vi "TEC Server.vi"() -> ()   [LabVIEW 2025]
uses:
  controls/TED4015 Connection.ctl
  controls/TED4015 Status.ctl
  <vilib>/Utility/error.llb/DialogType.ctl
  <vilib>/addons/_JKI Toolkits/State Machine/_JKI_lib_State_Machine.llb/Select State(s)_err__jki_lib_state_machine.vi
  <vilib>/addons/_JKI Toolkits/State Machine/_JKI_lib_State_Machine.llb/Periodic Trigger__ogtk__JKI-SM__jki_lib_state_machine.vi
  <userlib>/_OpenG.lib/comparison/comparison.llb/1D Boolean Array Changed__ogtk.vi
  <userlib>/_OpenG.lib/comparison/comparison.llb/openg_comparison__ogtk.lvlib
panel:
  in  "DiodeNames":string[](array[string])=["InAs", "InGaAs"]
  in  "DiodeNames 2":string[](array[string])
  out "error out":errorcluster {"code" format="%.0x"}
  in  "Tab Control":enum32{"Graph", "Export"}(tab)
  out "TED":waveform(dbl)[](graph)=[{"t0"=timestamp(3845871052.1406174 s since 1904-01-01), "dt"=1.0, "Y"=[23.85494], "attributes"=variant("NI_ChannelName"=variant(string "TED_Temp_0"))}, {"t0"=timestamp(3845871052.1406174 s since 1904-01-01), "dt"=1.0, "Y"=[0.0], "attributes"=variant("NI_ChannelName"=variant(string "TED_Voltage_0"))}, {"t0"=timestamp(3845871052.1406174 s since 1904-01-01), "dt"=1.0, "Y"=[0.001787742], "attributes"=variant("NI_ChannelName"=variant(string "TED_Current_0"))}, {"t0"=timestamp(3845871052.1406174 s since 1904-01-01), "dt"=1.0, "Y"=[21.97219], "attributes"=variant("NI_ChannelName"=variant(string "TED_Temp_1"))}, {"t0"=timestamp(3845871052.1406174 s since 1904-01-01), "dt"=1.0, "Y"=[0.0], "attributes"=variant("NI_ChannelName"=variant(string "TED_Voltage_1"))}, {"t0"=timestamp(3845871052.1406174 s since 1904-01-01), "dt"=1.0, "Y"=[0.00642528], "attributes"=variant("NI_ChannelName"=variant(string "TED_Current_1"))}]
  out "TED_Wfm":T1={"Temp"=[{"t0"=timestamp(3845871052.1406174 s since 1904-01-01), "dt"=1.0, "Y"=[23.85494], "attributes"=variant("NI_ChannelName"=variant(string "TED_Temp_0"))}, {"t0"=timestamp(3845871052.1406174 s since 1904-01-01), "dt"=1.0, "Y"=[21.97219], "attributes"=variant("NI_ChannelName"=variant(string "TED_Temp_1"))}], "Volts"=[{"t0"=timestamp(3845871052.1406174 s since 1904-01-01), "dt"=1.0, "Y"=[0.001787742], "attributes"=variant("NI_ChannelName"=variant(string "TED_Current_0"))}, {"t0"=timestamp(3845871052.1406174 s since 1904-01-01), "dt"=1.0, "Y"=[0.00642528], "attributes"=variant("NI_ChannelName"=variant(string "TED_Current_1"))}], "Amps"=[{"t0"=timestamp(3845871052.1406174 s since 1904-01-01), "dt"=1.0, "Y"=[0.0], "attributes"=variant("NI_ChannelName"=variant(string "TED_Voltage_0"))}, {"t0"=timestamp(3845871052.1406174 s since 1904-01-01), "dt"=1.0, "Y"=[0.0], "attributes"=variant("NI_ChannelName"=variant(string "TED_Voltage_1"))}]}
  in  "TEC On":bool[](array[boolean])=[FALSE, FALSE]
  in  "TED Status":T2[](array[typedef])=[{"Output"=FALSE, "SetPoint"=-65.00001, "Temperature"=23.85494, "Current"=0.0, "Voltage"=0.001787742, "CableTrip"=FALSE, "TransducerTrip"=FALSE, "OverTemp"=FALSE}, {"Output"=FALSE, "SetPoint"=-65.00001, "Temperature"=21.97219, "Current"=0.0, "Voltage"=0.00642528, "CableTrip"=FALSE, "TransducerTrip"=FALSE, "OverTemp"=FALSE}]
  in  "TED4015s":T3[](array[typedef])=[{"VISA resource name"="TED-1", "Connected"=FALSE, "Serial Number"=""}, {"VISA resource name"="TED-2", "Connected"=FALSE, "Serial Number"=""}]
  in  "Exit":bool
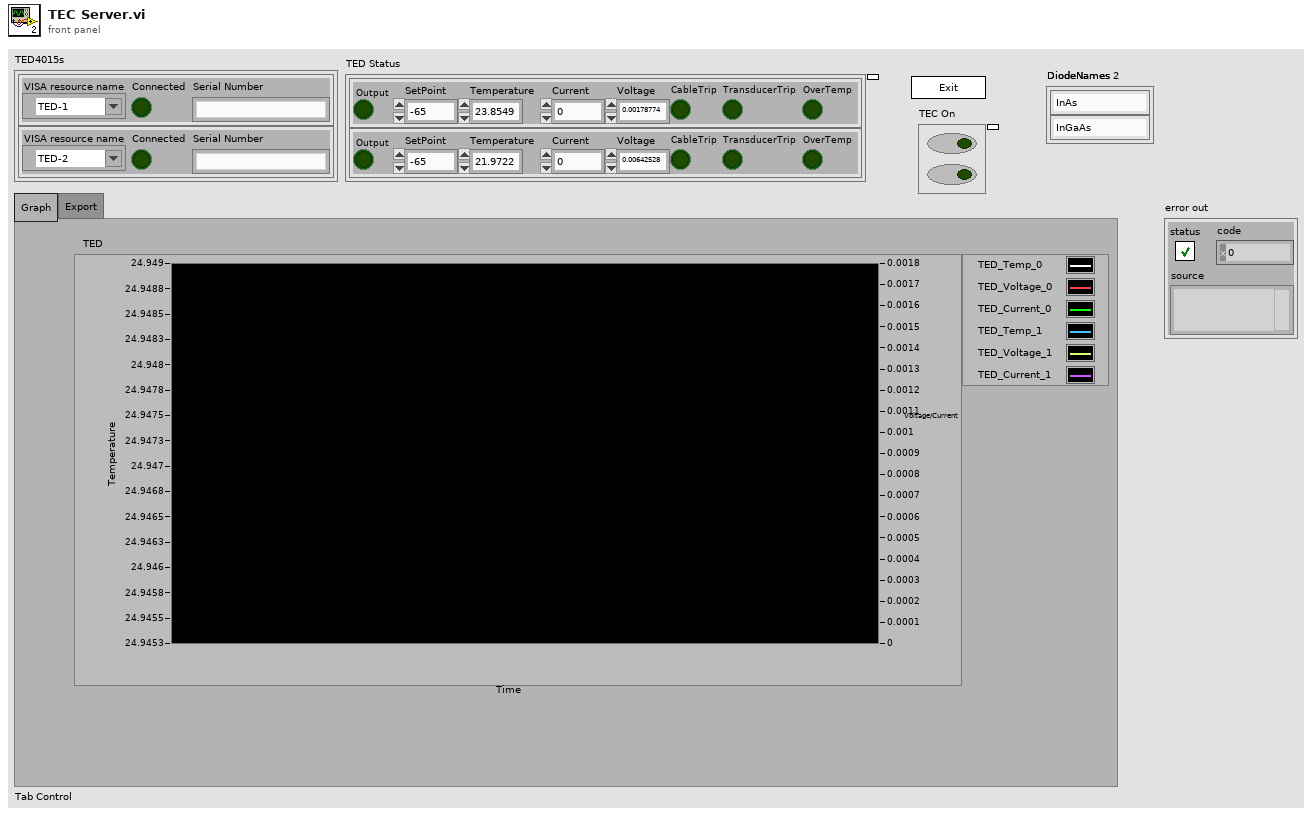
[diagram p1: front panel]
types:
  T1 = cluster{"Temp":waveform(dbl)[], "Volts":waveform(dbl)[], "Amps":waveform(dbl)[]}
  T2 = typedef "TED4015 Status.ctl" = cluster{"Output":bool, "SetPoint":dbl, "Temperature":dbl, "Current":dbl, "Voltage":dbl, "CableTrip":bool, "TransducerTrip":bool, "OverTemp":bool}
  T3 = typedef "TED4015 Connection.ctl" = cluster{"VISA resource name":refnum<visa-resource-name>, "Connected":bool, "Serial Number":string}
  T4 = enum32{"invalid app kind", "Development System", "Run Time System", "Student Edition", "Embedded LabVIEW", "Evaluation", "Custom"}
  T5 = enum32{"Invalid", "Standard", "Closed", "Hidden", "Minimized", "Maximized"}
  T6 = cluster{"Core":cluster{"Current VI Reference":refnum<vi>, "Close Panel on Exit?":bool}, "TED4015s":T3[], "TED Status":T2[], "TED_Wfm":cluster{"Temp":waveform(dbl)[], "Volts":waveform(dbl)[], "Amps":waveform(dbl)[]}}
  T7 = typedef "DialogType.ctl" = u16
  T8 = cluster{"Current VI Reference":refnum<vi>, "Close Panel on Exit?":bool}
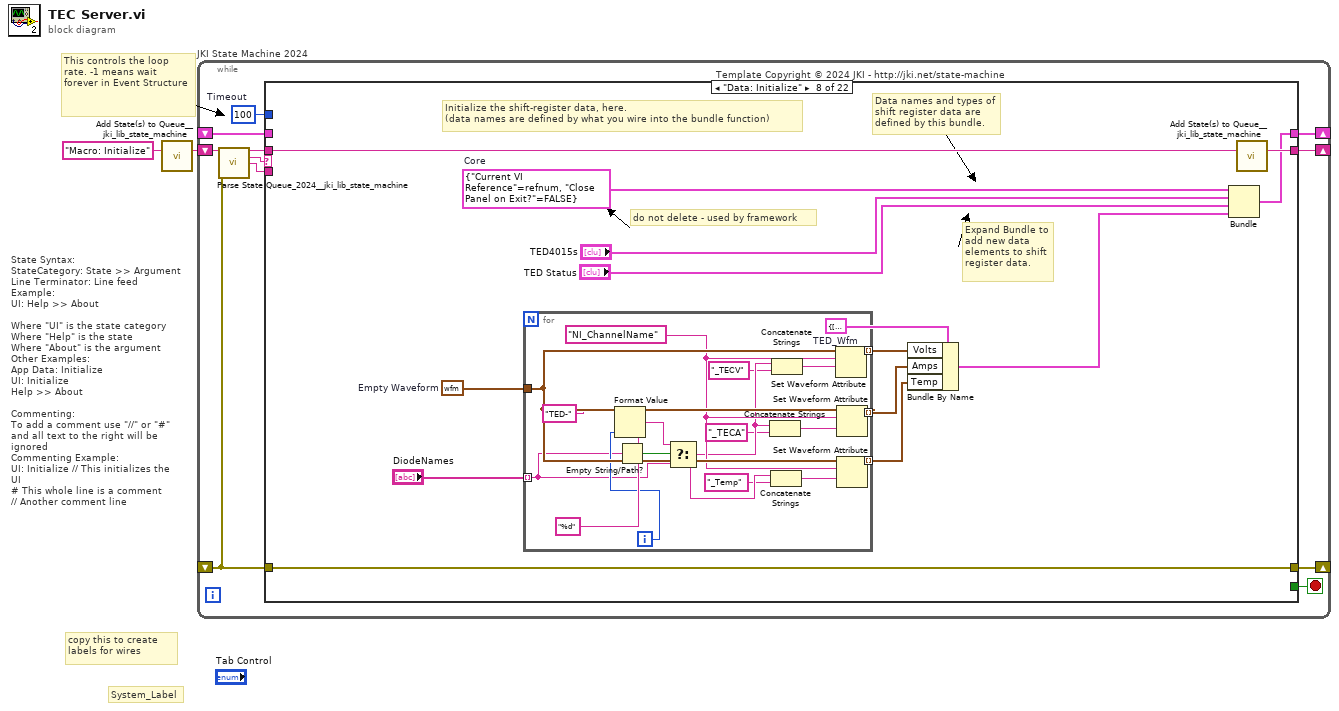
[diagram p0: block diagram]
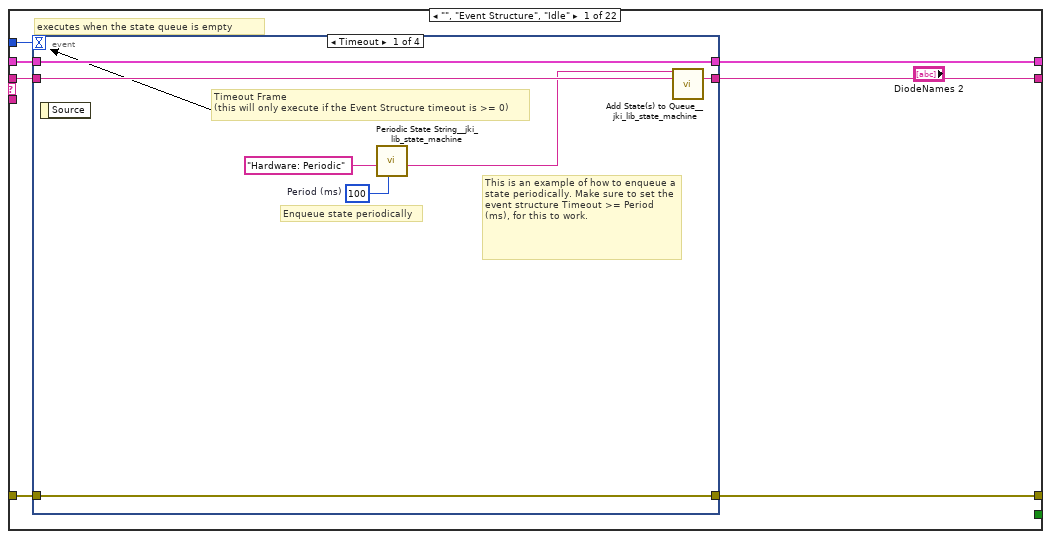
[diagram p2: hidden frame]
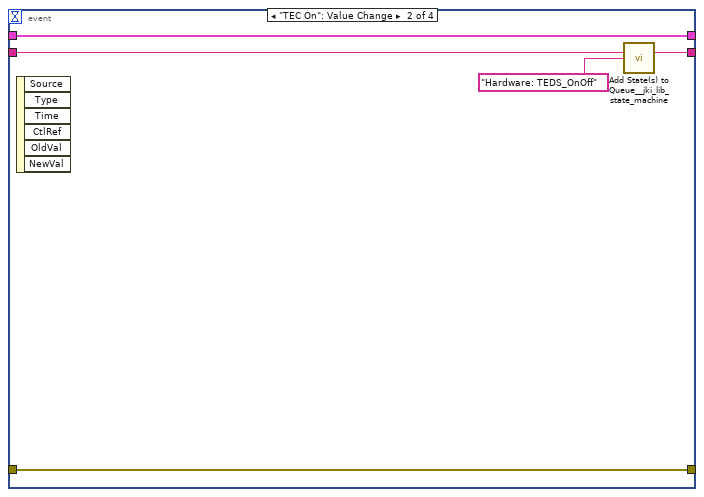
[diagram p3: hidden frame]
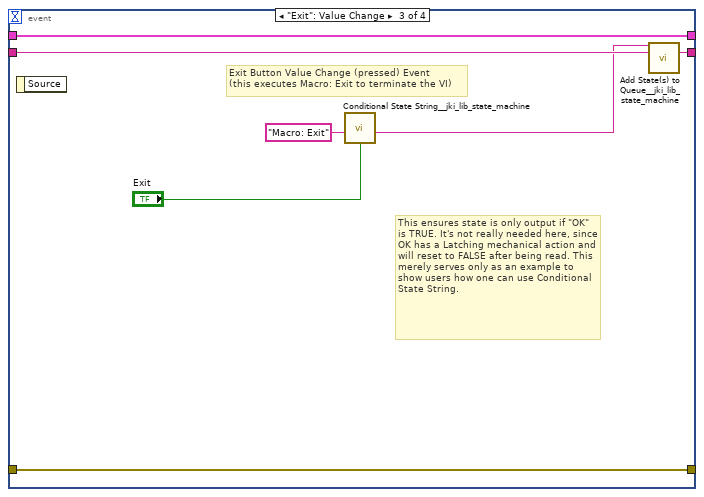
[diagram p4: hidden frame]
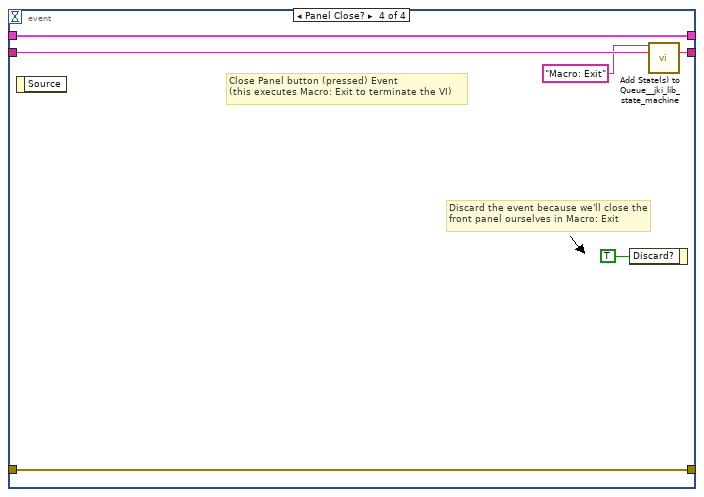
[diagram p5: hidden frame]
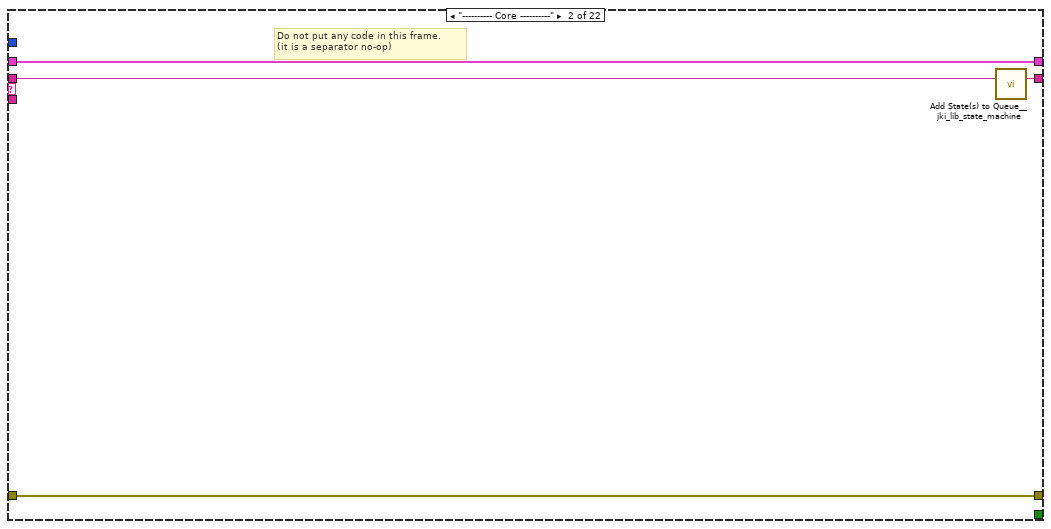
[diagram p6: hidden frame]
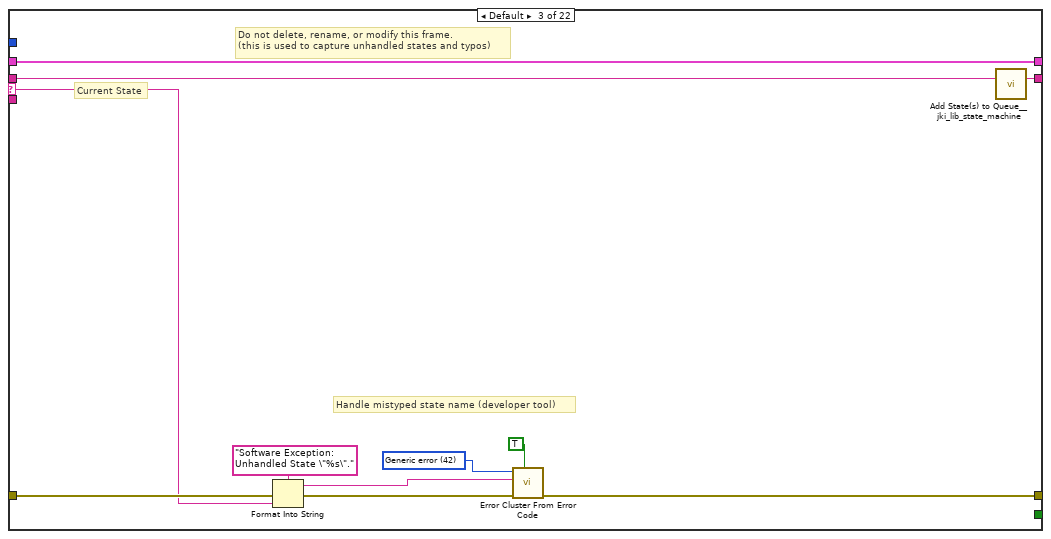
[diagram p7: hidden frame]
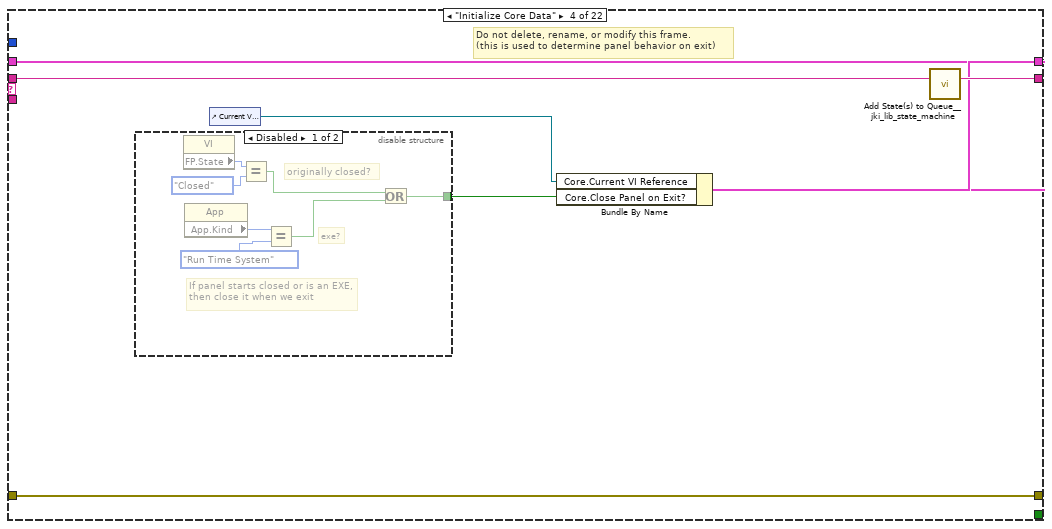
[diagram p8: hidden frame]
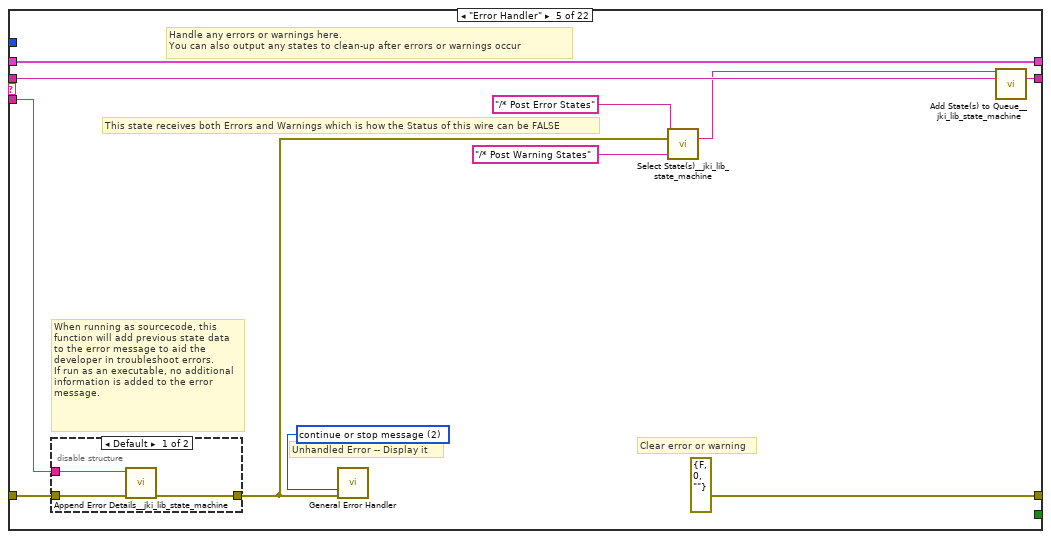
[diagram p10: hidden frame]
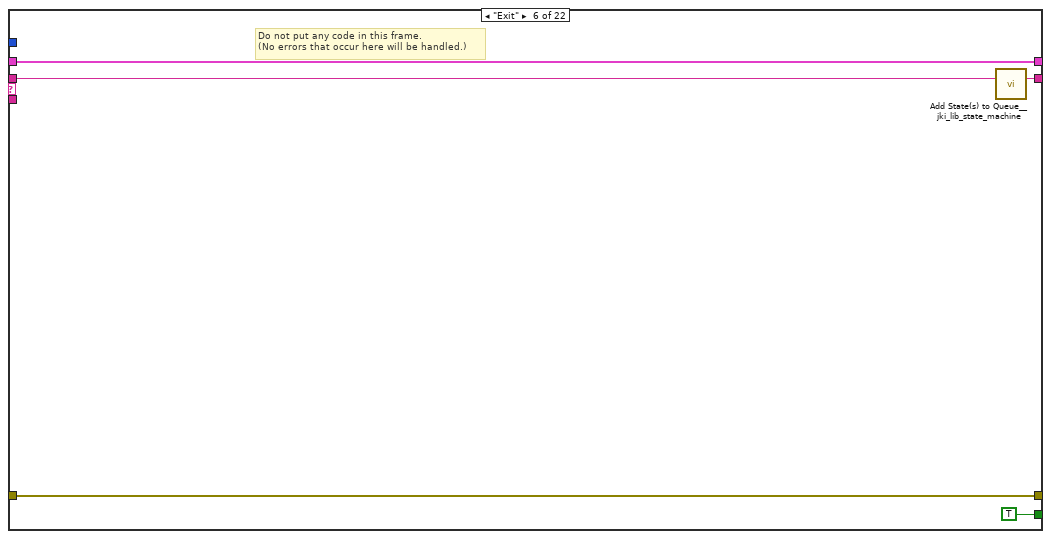
[diagram p12: hidden frame]
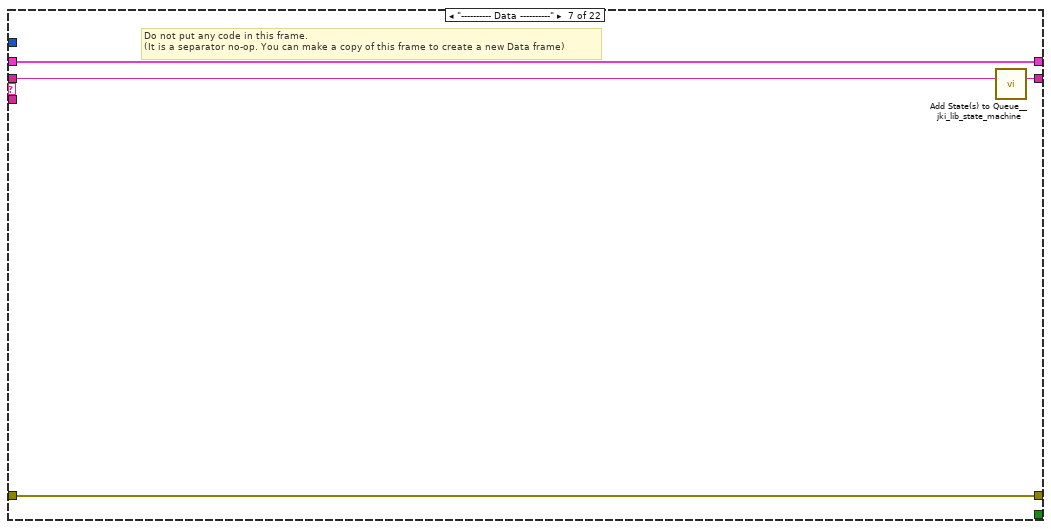
[diagram p13: hidden frame]
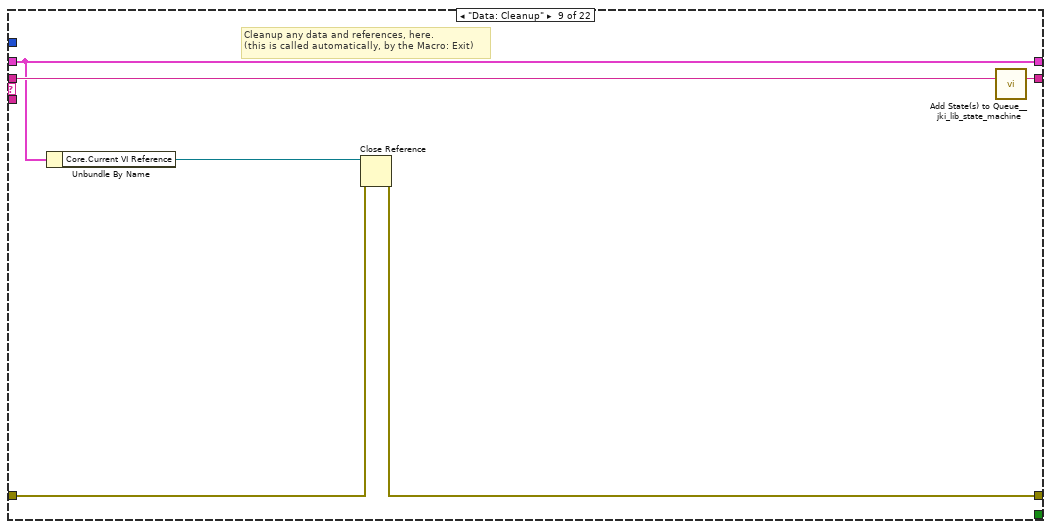
[diagram p14: hidden frame]
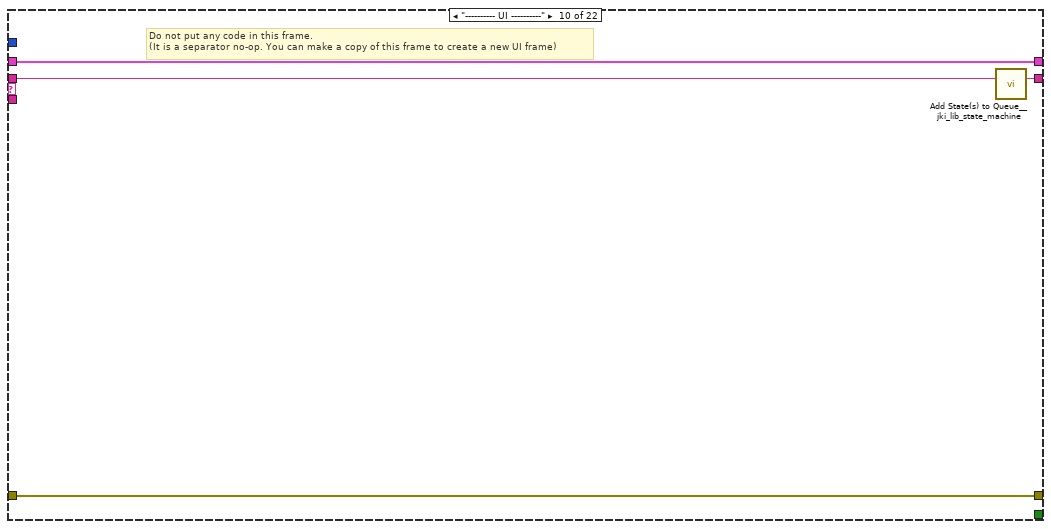
[diagram p15: hidden frame]
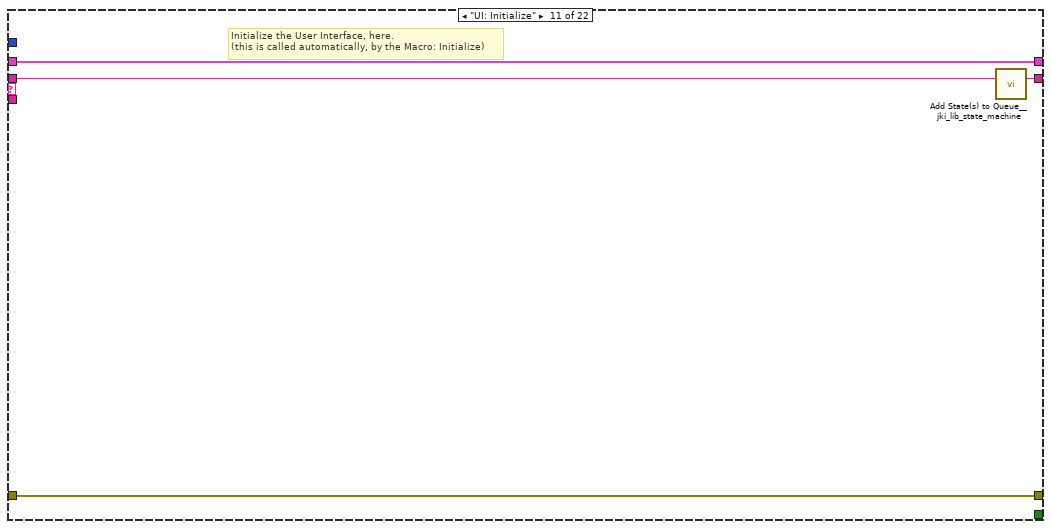
[diagram p16: hidden frame]
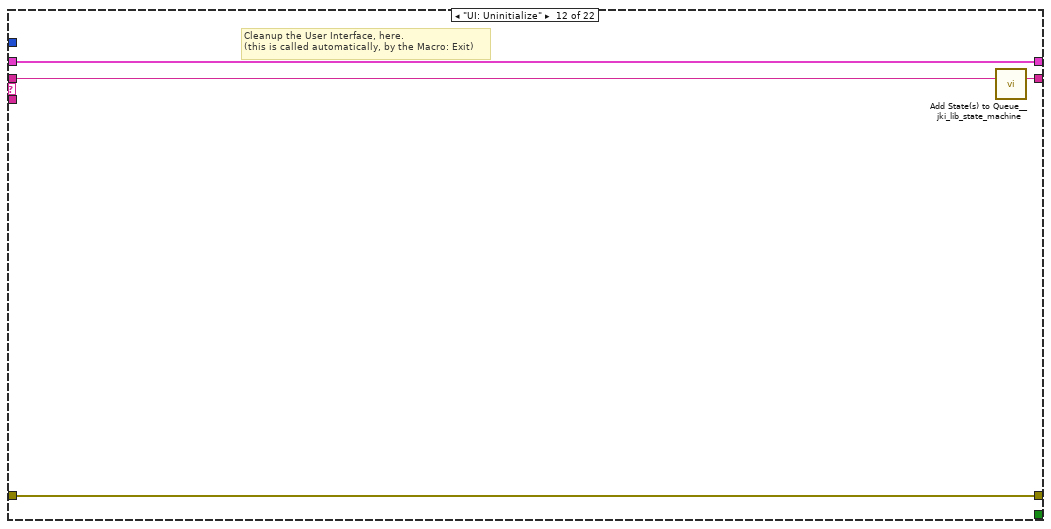
[diagram p17: hidden frame]
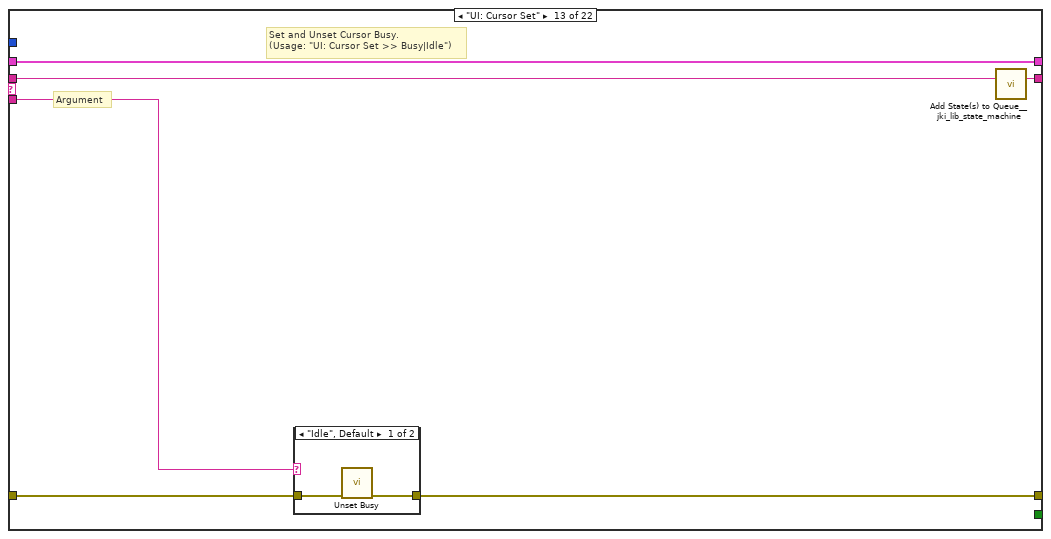
[diagram p18: hidden frame]
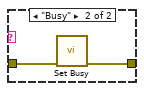
[diagram p19: hidden frame]
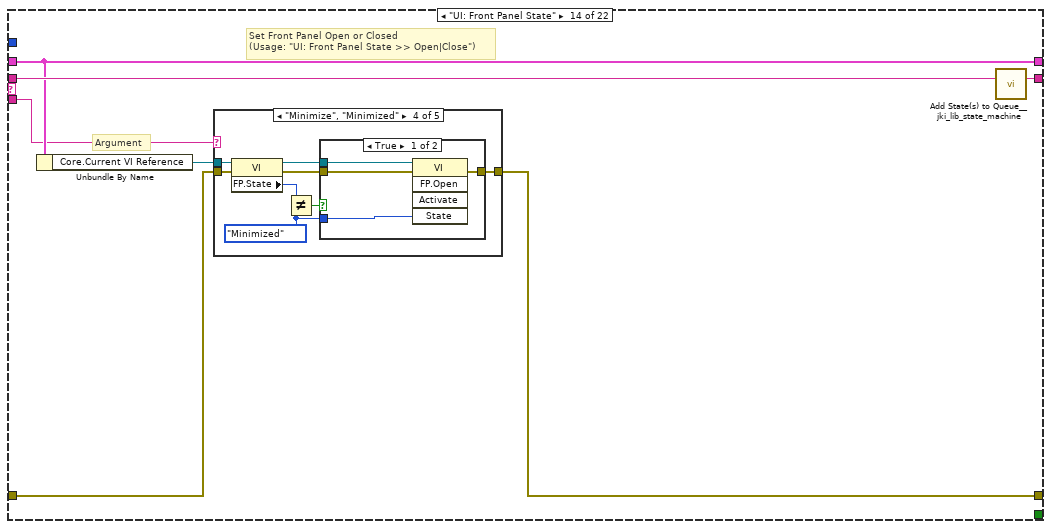
[diagram p20: hidden frame]
diagram:
  # "State Syntax:\nStateCategory: State >> Argument\nLine Terminator: Line feed\nExample:\nUI: Help >> About\n\nWhere \"UI\" is the state category\nWhere \"Help\" is the state\nWhere \"About\" is the argument\nOther Examples:\nApp Data: Initialize\nUI: Initialize\nHelp >> About\n\nCommenting:\nTo add a comment use \"//\" or \"#\" and all text to the right will be ignored\nCommenting Example:\nUI: Initialize // This initializes the UI\n# This whole line is a comment\n// Another comment line"
  # "copy this to create labels for wires"
  # "This controls the loop rate. -1 means wait forever in Event Structure"
  # "System_Label"
  n1 = call <vilib>:"Add State(s) to Queue__jki_lib_state_machine.vi"("State(s) in (\"\")"="Macro: Initialize") -> ("States Out"=w2:string)  [unwired: 14 in]
  n2 = while "JKI State Machine 2024" {
    shift-right: [w6] -> _
    shift-left: _ -> [w5]
    shift-right: [w9] -> _
    shift-left: _ -> [w3]
    shift-right: [w8] -> _
    shift-left: w2 -> [w10]
    stop <- w7 stop-if-true
    w4 = 100  # Timeout
    # "Template Copyright © 2024 JKI - http://jki.net/state-machine"
    n3 = call <vilib>:"Parse State Queue_2024__jki_lib_state_machine.vi"("State Queue"=w10, "Error In (no error)"=w3) -> ("Remaining States"=w12:string, "Current State"=w13:string, "Arguments"=w11:string)  [unwired: 11 in]
    n4 = case shown="\"Data: Initialize\"" w13 {
      selector: w13 -> [_ _ w50 _ _ _ _ _ _ _ _ _ _ _ _ _ _ _ _ _ _ _]
      tunnel: w12 -> [w20 w49 w54 w67 w85 w94 w98 w112 w136 w140 w144 w148 w154 w165 w234 w239 w248 w252 w260 w291 w316 w339]
      tunnel: w11 -> [_ _ _ _ w80 _ _ _ _ _ _ _ w149 w159 _ _ _ _ _ _ _ _]
      tunnel: w5 -> [w18 w46 w52 w63 w82 w92 w95 _ w131 w137 w142 w146 w152 w161 w231 w236 w246 w249 w258 w288 w306 w336]
      tunnel: [w17 w47 w56 w64 errorcluster {"status"=FALSE, "code"=0, "source"=""} ("error out") w91 w96 w109 w132 w138 w141 w145 w150 w162 w232 w237 w243 w250 w255 w285 w311 w333] -> w9
      tunnel: w3 -> [w14 w47 w55 w64 w81 w91 w96 w109 w133 w138 w141 w145 w151 w163 w232 w237 w243 w250 w256 w286 w312 w335]
      tunnel: [w19 w48 w53 w66 w84 w93 w97 w111 w135 w139 w143 w147 w153 w164 w233 w238 w247 w251 w259 w290 w315 w338] -> w8
      tunnel: [_ _ _ _ _ TRUE _ _ _ _ _ _ _ _ _ _ _ _ _ _ _ _] -> w7
      tunnel: [w16 w46 w52 w65 w82 w92 w95 w110 w131 w137 w142 w146 w152 w161 w231 w236 w246 w249 w254 w287 w313 w336] -> w6
      tunnel: w4 -> [w15 _ _ _ _ _ _ _ _ _ _ _ _ _ _ _ _ _ _ _ _ _]
      frame "", "Event Structure", "Idle" {
        # "executes when the state queue is empty"
        n5 = event shown="[0] Timeout" {
          selector: _ -> [_ _ _ _]
          dyn-events: _ -> [_ _ _ _]
          timeout: w15 -> [_ _ _ _]
          tunnel: w20 -> [w27 w30 w39 w45]
          tunnel: [w26 w31 w38 w44] -> w19
          tunnel: w18 -> [w24 w32 w36 w42]
          tunnel: [w25 w28 w37 w43] -> w17
          tunnel: w14 -> [w25 w28 w37 w43]
          tunnel: [w24 w32 w36 w42] -> w16
          event Timeout {
            w21 = u32 100  # Period (ms)
            # "Enqueue state periodically"
            # "This is an example of how to enqueue a state periodically. Make sure to set the event structure Timeout >= Period (ms), for this to work."
            # "Timeout Frame\n(this will only execute if the Event Structure timeout is >= 0)"
            n6 = event-data() -> ()  [unwired: 1 in, 1 out]
            n7 = call <vilib>:"Periodic State String__jki_lib_state_machine.vi"("Period (ms)"=w21, "State"="Hardware: Periodic") -> ("State Out"=w23:string)  [unwired: 9 in]
            n8 = call <vilib>:"Add State(s) to Queue__jki_lib_state_machine.vi"("State(s) in Front (\"\")"=w23, "State(s) in (\"\")"=w27) -> ("States Out"=w26:string)  [unwired: 13 in]
          }
          event "TEC On": Value Change {
            n9 = event-data() -> ()  [unwired: 1 in, 6 out]
            n10 = call <vilib>:"Add State(s) to Queue__jki_lib_state_machine.vi"("State(s) in (\"\")"=w30, "State(s) at Back (\"\")"="Hardware: TEDS_OnOff" ("State(s) at Back (\"\")")) -> ("States Out"=w31:string)  [unwired: 13 in]
          }
          event "Exit": Value Change {
            # "This ensures state is only output if \"OK\" is TRUE. It's not really needed here, since OK has a Latching mechanical action and will reset to FALSE after being read. This merely serves only as an example to show users how one can use Conditional State String."
            # "Exit Button Value Change (pressed) Event\n(this executes Macro: Exit to terminate the VI)"
            n11 = event-data() -> ()  [unwired: 1 in, 1 out]
            n12 = call <vilib>:"Conditional State String__jki_lib_state_machine.vi"("Do State(s)?"="Exit", "State"="Macro: Exit") -> ("State Out"=w33:string)  [unwired: 7 in]
            n13 = call <vilib>:"Add State(s) to Queue__jki_lib_state_machine.vi"("State(s) in Front (\"\")"=w33, "State(s) in (\"\")"=w39) -> ("States Out"=w38:string)  [unwired: 13 in]
          }
          event Panel Close? {
            # "Discard the event because we'll close the front panel ourselves in Macro: Exit"
            # "Close Panel button (pressed) Event\n(this executes Macro: Exit to terminate the VI)"
            n14 = event-data() -> ()  [unwired: 1 in, 1 out]
            n15 = event-data("Discard?"=TRUE) -> ()  [unwired: 1 in, 1 out]
            n16 = call <vilib>:"Add State(s) to Queue__jki_lib_state_machine.vi"("State(s) in Front (\"\")"="Macro: Exit", "State(s) in (\"\")"=w45) -> ("States Out"=w44:string)  [unwired: 13 in]
          }
        }
      }
      frame "---------- Core ----------" {
        # "Do not put any code in this frame.\n(it is a separator no-op)"
        n17 = call <vilib>:"Add State(s) to Queue__jki_lib_state_machine.vi"("State(s) in (\"\")"=w49) -> ("States Out"=w48:string)  [unwired: 14 in]
      }
      frame Default {
        w59 = 42 items=["No error", "Argument error", "Memory is full", "Out of zone", "End of file", "File already open", "Generic file I/O error", "File not found", "File permission error", "Disk is full", "Duplicate path", "Too many files open", "System feature not enabled", "Resource file not found", "Cannot add resource", "Resource not found", "Image not found", "Image memory error", "Pen does not exist", "Config type invalid", "Config token not found", "Config parse error", "Config memory error", "Bad external code format", "Bad external code offset", "External code not present", "Null window", "Destroy window error", "Null menu", "Print aborted", "Bad print record", "Print driver error", "Windows error during printing", "Memory error during printing", "Print dialog error", "Generic print error", "Invalid device refnum", "Device not found", "Device parameter error", "Device unit error", "Cannot open device", "Device call aborted", "Generic error", "Cancelled by user", "Object ID too low", "Object ID too high", "Object not in heap", "Unknown heap", "Unknown object (invalid DefProc)", "Unknown object (DefProc not in table)", "Message out of range", "Invalid (null) method", "Unknown message", "Manager call not supported", "Bad address", "Network operation in progress", "Network operation timed out", "Connection is busy", "Network attribute not supported", "Network error", "Address in use", "System out of memory", "Connection aborted", "Connection refused", "Not connected", "Already connected", "Connection closed", "Initialization error (interapplication manager)", "Bad occurrence", "Wait on unbound occurrence handler", "Occurrence queue overflow", "Datalog type conflict", "Unused", "Unrecognized type (interapplication manager)", "Memory corrupt", "Failed to make temporary DLL", "Old CIN version", "Drag socket not found", "Failed to load drop-object", "Failed to register OLE object", "Failed to release OLE object", "Format specifier type mismatch", "Unknown format specifier", "Too few format specifiers", "Too many format specifiers", "Scan failed", "Newer CIN version", "Error converting to variant", "Runtime menu error", "Password tampered", "Variant attribute not found", "Incompatible variant data type", "Event data is not available", "Event Store is not present", "Occurrence is not found", "Event Queue is not created", "Event info is not available", "Refnum passed is NULL", "Error retrieving Class GUID", "Error retrieving CoClass GUID", "Error retrieving TypeLib GUID.", "Bad built application magic bytes.", "Specific driver is different from the specific driver associated with the Logical Name.", "There is no session opened to the class driver.", "Max Error", "MAX - Error with config objects", "MAX - Error loading configuration", "MAX - Group not supported"]
        # "Current State"
        # "Do not delete, rename, or modify this frame.\n(this is used to capture unhandled states and typos)"
        # "Handle mistyped state name (developer tool)"
        n18 = Format Into String(format string="Software Exception: Unhandled State \"%s\"." ("message"), error in=w55, w50) -> (resulting string=w58:string, error out=w57:errorcluster)  [unwired: 1 in]
        n19 = call <vilib>:"Error Cluster From Error Code.vi"("show call chain? (False)"=TRUE, "error in (no error)"=w57, "error message (\"\")"=w58, "error code (0)"=w59) -> ("error out"=w56:errorcluster)  [unwired: 5 in]
        n20 = call <vilib>:"Add State(s) to Queue__jki_lib_state_machine.vi"("State(s) in (\"\")"=w54) -> ("States Out"=w53:string)  [unwired: 14 in]
      }
      frame "Initialize Core Data" {
        # "Do not delete, rename, or modify this frame.\n(this is used to determine panel behavior on exit)"
        n21 = disable-structure shown="Disabled" {
          disable-tunnel: [w74 _] -> w61
          frame Disabled {
            # "originally closed?"
            # "If panel starts closed or is an EXE, then close it when we exit"
            # "exe?"
            n22 = property class="VI"() -> ("FP.State"=w71:T5)  [unwired: 2 in, 2 out]
            n23 = property class="App"() -> ("App.Kind"=w68:T4)  [unwired: 2 in, 2 out]
            n24 = Equal?(x=w71, y=T5."Closed" ("Front Panel Window:State")) -> (x = y?=w73:bool)
            n25 = Equal?(x=w68, y=T4."Run Time System" ("Application:Kind")) -> (x = y?=w70:bool)
            n26 = Or(x=w73, y=w70) -> (x .or. y?=w74:bool)
          }
          frame Enabled {
          }
        }
        n27 = control-ref of="Current VI Reference"() -> (w62:refnum<vi>)
        n28 = Bundle By Name(cluster=w63, "Core.Current VI Reference"=w62, "Core.Close Panel on Exit?"=w61) -> (w65:T6)
        n29 = call <vilib>:"Add State(s) to Queue__jki_lib_state_machine.vi"("State(s) in (\"\")"=w67) -> ("States Out"=w66:string)  [unwired: 14 in]
      }
      frame "Error Handler" {
        w75 = T7 2 items=["no dialog", "OK message", "continue or stop message", "OK message + warnings", "continue/stop + warnings"] ("type of dialog (OK msg:1)")
        # "When running as sourcecode, this function will add previous state data to the error message to aid the developer in troubleshoot errors.\nIf run as an executable, no additional information is added to the error message."
        # "This state receives both Errors and Warnings which is how the Status of this wire can be FALSE"
        # "Unhandled Error -- Display it"
        # "Handle any errors or warnings here.\nYou can also output any states to clean-up after errors or warnings occur"
        # "Clear error or warning"
        n30 = disable-structure shown="Default" {
          disable-tunnel: w81 -> [w88 w89]
          disable-tunnel: w80 -> [w87 _]
          disable-tunnel: [w86 w89] -> w79
          frame condition #0 (active) {
            n31 = call <vilib>:"Append Error Details__jki_lib_state_machine.vi"("error in (no error)"=w88, "Previous State and Argument(s)"=w87) -> ("error out"=w86:errorcluster)  [unwired: 9 in]
          }
          frame condition #1 {
          }
        }
        n32 = call <vilib>:"General Error Handler.vi"("type of dialog (OK msg:1)"=w75, "error in (no error)"=w79) -> ()  [unwired: 9 in, 5 out]
        n33 = call-poly <vilib>:"Select State(s)__jki_lib_state_machine.vi"("State(s) if True (\"\")"="/* Post Error States", "Select"=w79, "State(s) if False (\"\")"="/* Post Warning States") -> ("States Out"=w77:string)  [unwired: 12 in]
        n34 = call <vilib>:"Add State(s) to Queue__jki_lib_state_machine.vi"("State(s) in Front (\"\")"=w77, "State(s) in (\"\")"=w85) -> ("States Out"=w84:string)  [unwired: 13 in]
      }
      frame "Exit" {
        # "Do not put any code in this frame.\n(No errors that occur here will be handled.)"
        n35 = call <vilib>:"Add State(s) to Queue__jki_lib_state_machine.vi"("State(s) in (\"\")"=w94) -> ("States Out"=w93:string)  [unwired: 14 in]
      }
      frame "---------- Data ----------" {
        # "Do not put any code in this frame.\n(It is a separator no-op. You can make a copy of this frame to create a new Data frame)"
        n36 = call <vilib>:"Add State(s) to Queue__jki_lib_state_machine.vi"("State(s) in (\"\")"=w98) -> ("States Out"=w97:string)  [unwired: 14 in]
      }
      frame "Data: Initialize" {
        w104 = T1 {"Temp"=[], "Volts"=[], "Amps"=[]}  # TED_Wfm
        w105 = waveform(dbl) {"t0"=timestamp(0 s since 1904-01-01), "dt"=1.0, "Y"=[]}  # Empty Waveform
        w108 = T8 {"Current VI Reference"=refnum, "Close Panel on Exit?"=FALSE}  # Core
        # "do not delete - used by framework"
        # "Expand Bundle to add new data elements to shift register data."
        # "Data names and types of shift register data are defined by this bundle."
        # "Initialize the shift-register data, here.\n(data names are defined by what you wire into the bundle function)"
        n37 = for {
          tunnel: w105 -> [w129]
          tunnel: [w128] -> w103 mode=indexing
          tunnel: [w127] -> w102 mode=indexing
          tunnel: [w126] -> w101 mode=indexing
          tunnel: "DiodeNames" -> [w119] mode=indexing
          i -> [w124]
          w125 = "NI_ChannelName" ("name")
          n38 = Format Value(string ("")="TED-", format string="%d", value (0)=w124) -> (output string=w118:string)
          n39 = Empty String/Path?(string/path=w119) -> (empty?=w120:bool)
          n40 = Select(t=w118, s=w120, f=w119) -> (s? t:f=w121:string)
          n41 = Concatenate Strings(w121, "_TECA" ("string")) -> (w115:string)
          n42 = Concatenate Strings(w121, "_Temp" ("string")) -> (w117:string)
          n43 = Concatenate Strings(w121, "_TECV" ("string")) -> (w122:string)
          n44 = Set Waveform Attribute(5:w122, 6:w125, 7:w129) -> (3:w128:waveform(dbl))  [unwired: 1 in, 2 out]
          n45 = Set Waveform Attribute(5:w115, 6:w125, 7:w129) -> (3:w127:waveform(dbl))  [unwired: 1 in, 2 out]
          n46 = Set Waveform Attribute(5:w117, 6:w125, 7:w129) -> (3:w126:waveform(dbl))  [unwired: 1 in, 2 out]
        }
        n47 = Bundle By Name(cluster=w104, "Volts"=w103, "Amps"=w102, "Temp"=w101) -> (w100:T1)
        n48 = Bundle("Core"=w108, "TED4015s"="TED4015s", "TED Status"="TED Status", "TED_Wfm"=w100) -> (w110:T6)  [unwired: 1 in]
        n49 = call <vilib>:"Add State(s) to Queue__jki_lib_state_machine.vi"("State(s) in (\"\")"=w112) -> ("States Out"=w111:string)  [unwired: 14 in]
      }
      frame "Data: Cleanup" {
        # "Cleanup any data and references, here.\n(this is called automatically, by the Macro: Exit)"
        n50 = Unbundle By Name(w131) -> ("Core.Current VI Reference"=w134:refnum<vi>)
        n51 = Close Reference(reference=w134, error in (no error)=w133) -> (error out=w132:errorcluster)
        n52 = call <vilib>:"Add State(s) to Queue__jki_lib_state_machine.vi"("State(s) in (\"\")"=w136) -> ("States Out"=w135:string)  [unwired: 14 in]
      }
      frame "---------- UI ----------" {
        # "Do not put any code in this frame.\n(It is a separator no-op. You can make a copy of this frame to create a new UI frame)"
        n53 = call <vilib>:"Add State(s) to Queue__jki_lib_state_machine.vi"("State(s) in (\"\")"=w140) -> ("States Out"=w139:string)  [unwired: 14 in]
      }
      frame "UI: Initialize" {
        # "Initialize the User Interface, here.\n(this is called automatically, by the Macro: Initialize)"
        n54 = call <vilib>:"Add State(s) to Queue__jki_lib_state_machine.vi"("State(s) in (\"\")"=w144) -> ("States Out"=w143:string)  [unwired: 14 in]
      }
      frame "UI: Uninitialize" {
        # "Cleanup the User Interface, here.\n(this is called automatically, by the Macro: Exit)"
        n55 = call <vilib>:"Add State(s) to Queue__jki_lib_state_machine.vi"("State(s) in (\"\")"=w148) -> ("States Out"=w147:string)  [unwired: 14 in]
      }
      frame "UI: Cursor Set" {
        # "Argument"
        # "Set and Unset Cursor Busy.\n(Usage: \"UI: Cursor Set >> Busy|Idle\")"
        n56 = case shown="\"Idle\", Default" w149 {
          tunnel: w151 -> [w156 w158]
          tunnel: [w155 w157] -> w150
          frame "Idle", Default {
            n57 = call <vilib>:"Unset Busy.vi"("error in (no error)"=w156) -> ("error out"=w155:errorcluster)  [unwired: 10 in]
          }
          frame "Busy" {
            n58 = call <vilib>:"Set Busy.vi"("error in (no error)"=w158) -> ("error out"=w157:errorcluster)  [unwired: 9 in, 1 out]
          }
        }
        n59 = call <vilib>:"Add State(s) to Queue__jki_lib_state_machine.vi"("State(s) in (\"\")"=w154) -> ("States Out"=w153:string)  [unwired: 14 in]
      }
      frame "UI: Front Panel State" {
        # "Argument"
        # "Set Front Panel Open or Closed\n(Usage: \"UI: Front Panel State >> Open|Close\")"
        n60 = Unbundle By Name(w161) -> ("Core.Current VI Reference"=w160:refnum<vi>)
        n61 = case shown="\"Minimize\", \"Minimized\"" w159 {
          tunnel: w163 -> [w171 w186 w197 w210 w223]
          tunnel: [w173 w187 w199 w212 w225] -> w162
          tunnel: w160 -> [w172 w184 w198 w211 w224]
          frame "Open", "Standard", Default {
            w166 = T5."Standard" ("State")
            n62 = property class="VI"(reference=w172, error in=w171) -> (reference out=w169:refnum<vi>, error out=w170:errorcluster, "FP.State"=w168:T5)
            n63 = Not Equal?(x=w168, y=w166) -> (x != y?=w167:bool)
            n64 = case shown="True" w167 {
              tunnel: [w177 w179] -> w173
              tunnel: w170 -> [w176 w179]
              tunnel: w169 -> [w175 _]
              tunnel: w166 -> [w174 _]
              frame True {
                n65 = invoke class="VI" method="FP.Open"(reference=w175, error in=w176, "Activate"=TRUE, "State"=w174) -> (error out=w177:errorcluster)  [unwired: 1 in, 4 out]
              }
              frame False {
              }
            }
          }
          frame "Close", "Closed" {
            n66 = property class="VI"(reference=w184, error in=w186) -> (reference out=w183:refnum<vi>, error out=w185:errorcluster, "FP.State"=w181:T5)
            n67 = Not Equal?(x=w181, y=T5."Closed" ("Front Panel Window:State")) -> (x != y?=w180:bool)
            n68 = case shown="True" w180 {
              tunnel: [w188 w191] -> w187
              tunnel: w185 -> [w188 w190]
              tunnel: w183 -> [_ w189]
              frame False {
              }
              frame True {
                n69 = invoke class="VI" method="FP.Close"(reference=w189, error in=w190) -> (error out=w191:errorcluster)  [unwired: 1 in, 2 out]
              }
            }
          }
          frame "Hidden", "Hide" {
            w192 = T5."Hidden" ("State")
            n70 = property class="VI"(reference=w198, error in=w197) -> (reference out=w195:refnum<vi>, error out=w196:errorcluster, "FP.State"=w194:T5)
            n71 = Not Equal?(x=w194, y=w192) -> (x != y?=w193:bool)
            n72 = case shown="True" w193 {
              tunnel: [w203 w204] -> w199
              tunnel: w196 -> [w202 w204]
              tunnel: w195 -> [w201 _]
              tunnel: w192 -> [w200 _]
              frame True {
                n73 = invoke class="VI" method="FP.Open"(reference=w201, error in=w202, "State"=w200) -> (error out=w203:errorcluster)  [unwired: 2 in, 4 out]
              }
              frame False {
              }
            }
          }
          frame "Minimize", "Minimized" {
            w205 = T5."Minimized" ("State")
            n74 = property class="VI"(reference=w211, error in=w210) -> (reference out=w208:refnum<vi>, error out=w209:errorcluster, "FP.State"=w207:T5)
            n75 = Not Equal?(x=w207, y=w205) -> (x != y?=w206:bool)
            n76 = case shown="True" w206 {
              tunnel: [w216 w217] -> w212
              tunnel: w209 -> [w215 w217]
              tunnel: w208 -> [w214 _]
              tunnel: w205 -> [w213 _]
              frame True {
                n77 = invoke class="VI" method="FP.Open"(reference=w214, error in=w215, "State"=w213) -> (error out=w216:errorcluster)  [unwired: 2 in, 4 out]
              }
              frame False {
              }
            }
          }
          frame "Maximize", "Maximized" {
            w218 = T5."Maximized" ("State")
            n78 = property class="VI"(reference=w224, error in=w223) -> (reference out=w221:refnum<vi>, error out=w222:errorcluster, "FP.State"=w220:T5)
            n79 = Not Equal?(x=w220, y=w218) -> (x != y?=w219:bool)
            n80 = case shown="True" w219 {
              tunnel: [w229 w230] -> w225
              tunnel: w222 -> [w228 w230]
              tunnel: w221 -> [w227 _]
              tunnel: w218 -> [w226 _]
              frame True {
                n81 = invoke class="VI" method="FP.Open"(reference=w227, error in=w228, "State"=w226) -> (error out=w229:errorcluster)  [unwired: 2 in, 4 out]
              }
              frame False {
              }
            }
          }
        }
        n82 = call <vilib>:"Add State(s) to Queue__jki_lib_state_machine.vi"("State(s) in (\"\")"=w165) -> ("States Out"=w164:string)  [unwired: 14 in]
      }
      frame "---------- Macro ----------" {
        # "Do not put any code in this frame.\n(It is a separator no-op. You can make a copy of this frame to create a new Macro frame)"
        n83 = call <vilib>:"Add State(s) to Queue__jki_lib_state_machine.vi"("State(s) in (\"\")"=w234) -> ("States Out"=w233:string)  [unwired: 14 in]
      }
      frame "Macro: Initialize" {
        w235 = "Data: Initialize\nInitialize Core Data\nHardware: Initialise\nUI: Initialize\nUI: Front Panel State >> Open"  # Data: Initialize Initialize Core Data Hardware: Initialise UI: Initialize UI: Front Panel State >> Open
        # "Initialization Macro\n(This is called once, when the VI starts)"
        n84 = call <vilib>:"Add State(s) to Queue__jki_lib_state_machine.vi"("State(s) in Front (\"\")"=w235, "State(s) in (\"\")"=w239) -> ("States Out"=w238:string)  [unwired: 13 in]
      }
      frame "Macro: Exit" {
        # "Exit Macro\n(This is called once, when the VI exits)"
        n85 = Unbundle By Name(w246) -> ("Core.Close Panel on Exit?"=w241:bool)
        n86 = call <vilib>:"Conditional State String__jki_lib_state_machine.vi"("Do State(s)?"=w241, "State"="UI: Front Panel State >> Close") -> ("State Out"=w240:string)  [unwired: 7 in]
        n87 = call <vilib>:"Add State(s) to Queue__jki_lib_state_machine.vi"("State(s) in (\"\")"=w240, "State(s) at Back (\"\")"="Hardware: Cleanup\nUI: Uninitialize\nData: Cleanup\nExit") -> ("States Out"=w244:string)  [unwired: 13 in]
        n88 = call <vilib>:"Add State(s) to Queue__jki_lib_state_machine.vi"("State(s) in Front (\"\")"=w244, "State(s) in (\"\")"=w248) -> ("States Out"=w247:string)  [unwired: 13 in]
      }
      frame "---------- Hardware ----------" {
        # "Template Separator\n(You can make a copy of, or modify, this frame)"
        n89 = call <vilib>:"Add State(s) to Queue__jki_lib_state_machine.vi"("State(s) in (\"\")"=w252) -> ("States Out"=w251:string)  [unwired: 14 in]
      }
      frame "Hardware: Initialise" {
        # "Attempt to initialise each of the TED4015s and return serial numbers"
        n90 = Unbundle By Name(w258) -> ("TED4015s"=w257:T3[])
        n91 = for {
          tunnel: w257 -> [w264] mode=indexing
          tunnel: w256 -> [w265]
          tunnel: [w262] -> w255
          tunnel: [w261] -> w253 mode=indexing
          n92 = Unbundle By Name(w264) -> ("VISA resource name"=w266:refnum<visa-resource-name>)
          n93 = Empty String/Path?(string/path=w266) -> (empty?=w267:bool)
          n94 = case shown="False" w267 {
            tunnel: w266 -> [w281 _]
            tunnel: w265 -> [w280 w283]
            tunnel: [w277 w283] -> w262
            tunnel: [w276 ""] -> w263
            frame False {
              n95 = call <instrlib>:"TL4000 Initialize.vi"("error in (no error)"=w280, "resource name"=w281) -> ("error out"=w279:errorcluster, "instrument handle out"=w278:refnum<visa-resource-name>)  [unwired: 8 in]
              n96 = call <instrlib>:"TL4000 Identification Query.vi"("error in (no error)"=w279, "instrument handle"=w278) -> ("error out"=w277:errorcluster, "Serial Number"=w276:string)  [unwired: 4 in, 4 out]
            }
            frame True {
            }
          }
          n97 = case shown="Error .." w262 {
            tunnel: w264 -> [w271 w275]
            tunnel: w263 -> [w270 _]
            tunnel: [w269 w274] -> w261
            frame No Error {
              n98 = Bundle By Name(cluster=w271, "Connected"=TRUE, "Serial Number"=w270) -> (w269:T3)
            }
            frame Error {
              n99 = Bundle By Name(cluster=w275, "Connected"=FALSE, "Serial Number"="") -> (w274:T3)
            }
          }
        }
        n100 = Bundle By Name(cluster=w258, "TED4015s"=w253) -> (w254:T6)
        n101 = local write "TED4015s"(w253) -> ()
        n102 = call <vilib>:"Add State(s) to Queue__jki_lib_state_machine.vi"("State(s) in (\"\")"=w260) -> ("States Out"=w259:string)  [unwired: 14 in]
      }
      frame "Hardware: Cleanup" {
        # "Close both TED4015s"
        n103 = Unbundle By Name(w288) -> ("TED4015s"=w289:T3[])
        n104 = for {
          tunnel: w289 -> [w296] mode=indexing
          tunnel: w286 -> [w297]
          tunnel: [w295] -> w285
          tunnel: [w294] -> w284 mode=indexing
          n105 = Unbundle By Name(w296) -> ("VISA resource name"=w298:refnum<visa-resource-name>)
          n106 = Empty String/Path?(string/path=w298) -> (empty?=w299:bool)
          n107 = case shown="True" w299 {
            tunnel: w298 -> [_ w303]
            tunnel: w297 -> [w300 w302]
            tunnel: [w300 w301] -> w295
            frame False {
            }
            frame True {
              n108 = call <instrlib>:"TL4000 Close.vi"("error in (no error)"=w302, "instrument handle"=w303) -> ("error out"=w301:errorcluster)  [unwired: 9 in]
            }
          }
          n109 = Bundle By Name(cluster=w296, "Connected"=FALSE, "Serial Number"="") -> (w294:T3)
        }
        n110 = Bundle By Name(cluster=w288, "TED4015s"=w284) -> (w287:T6)
        n111 = local write "TED4015s"(w284) -> ()
        n112 = call <vilib>:"Add State(s) to Queue__jki_lib_state_machine.vi"("State(s) in (\"\")"=w291) -> ("States Out"=w290:string)  [unwired: 14 in]
      }
      frame "Hardware: Periodic" {
        # "Get status and other info from TEDs"
        n113 = Unbundle By Name(w306) -> ("TED4015s"=w314:T3[])
        n114 = for {
          tunnel: w314 -> [w325] mode=indexing
          tunnel: w312 -> [w326]
          tunnel: [w324] -> w311
          tunnel: [w321] -> w305 mode=indexing
          n115 = Unbundle By Name(w325) -> ("Connected"=w323:bool, "VISA resource name"=w322:refnum<visa-resource-name>)
          n116 = case shown="False" w323 {
            tunnel: w326 -> [w328 w332]
            tunnel: [w328 w331] -> w324
            tunnel: w322 -> [_ w330]
            tunnel: [w327 w329] -> w321
            frame False {
              w327 = T2 {"Output"=FALSE, "SetPoint"=nan, "Temperature"=nan, "Current"=nan, "Voltage"=nan, "CableTrip"=FALSE, "TransducerTrip"=FALSE, "OverTemp"=FALSE}  # NullTedStatus
            }
            frame True {
              n117 = call "get TED_Status.vi"("error in (no error)"=w332, "TED-VISA In"=w330) -> ("error out"=w331:errorcluster, "TED Status"=w329:T2)  [unwired: 7 in, 1 out]
            }
          }
        }
        n118 = in-place {
          in-place-border: w305 -> [w319]
          n119 = in-place-cluster #1(w306) -> ("TED_Wfm"=w320:T1)
          n120 = call "ConvertTEDtoWFM.vi"("TED Status"=w319, "Input cluster"=w320) -> ("TED"=→"TED":waveform(dbl)[], "TED_Wfm"=w318:T1)  [unwired: 8 in]
          "TED_Wfm" <- w318
          n121 = in-place-cluster #1("TED_Wfm"=w318) -> (w304:T6)
        }
        n122 = local write "TED Status"(w305) -> ()
        n123 = Bundle By Name(cluster=w304, "TED Status"=w305) -> (w313:T6)
        n124 = local read "TEC On"() -> (w310:bool[])
        n125 = call-poly <userlib>:"Data Changed__ogtk.vi"("1D Boolean Array"=w310) -> ("Changed"=w309:bool)
        n126 = call <vilib>:"Conditional State String__jki_lib_state_machine.vi"("Do State(s)?"=w309, "State"="Hardware: TEDS_OnOff") -> ("State Out"=w308:string)  [unwired: 7 in]
        n127 = call <vilib>:"Add State(s) to Queue__jki_lib_state_machine.vi"("State(s) in (\"\")"=w316, "State(s) at Back (\"\")"=w308) -> ("States Out"=w315:string)  [unwired: 13 in]
      }
      frame "Hardware: TEDS_OnOff" {
        # "Get status and other info from TEDs"
        n128 = Unbundle By Name(w336) -> ("TED4015s"=w337:T3[])
        n129 = for {
          tunnel: w337 -> [w344] mode=indexing
          tunnel: w335 -> [w345]
          tunnel: "TEC On" -> [w341] mode=indexing
          tunnel: [w340] -> w333
          n130 = Unbundle By Name(w344) -> ("Connected"=w343:bool, "VISA resource name"=w342:refnum<visa-resource-name>)
          n131 = case shown="True" w343 {
            tunnel: w345 -> [w346 w351]
            tunnel: [w346 w347] -> w340
            tunnel: w342 -> [_ w350]
            tunnel: w341 -> [_ w349]
            frame False {
            }
            frame True {
              n132 = call "TL4000 Switch TEC Output.vi"("error in (no error)"=w351, "TEC Output (Off)"=w349, "instrument handle"=w350) -> ("error out"=w348:errorcluster)  [unwired: 7 in, 1 out]
              "error out" <- w348
              n133 = call <vilib>:"Clear Errors.vi"("error in (no error)"=w348) -> ("error out"=w347:errorcluster)  [unwired: 5 in, 1 out]
            }
          }
        }
        n134 = call <vilib>:"Add State(s) to Queue__jki_lib_state_machine.vi"("State(s) in (\"\")"=w339) -> ("States Out"=w338:string)  [unwired: 14 in]
      }
    }
  }
